vi "Analog Parse Configuration Parameters.vi"(10 "Analog Configuration Parameters":T1) -> (0 "name to assign":string, 1 "physical channels":string, 3 "Maximum Voltage":dbl, 5 "Minimum Voltage":dbl, 7 "Terminal Configuration":i32)   [LabVIEW 2021]
uses:
  Analog Configuration Parameters.ctl
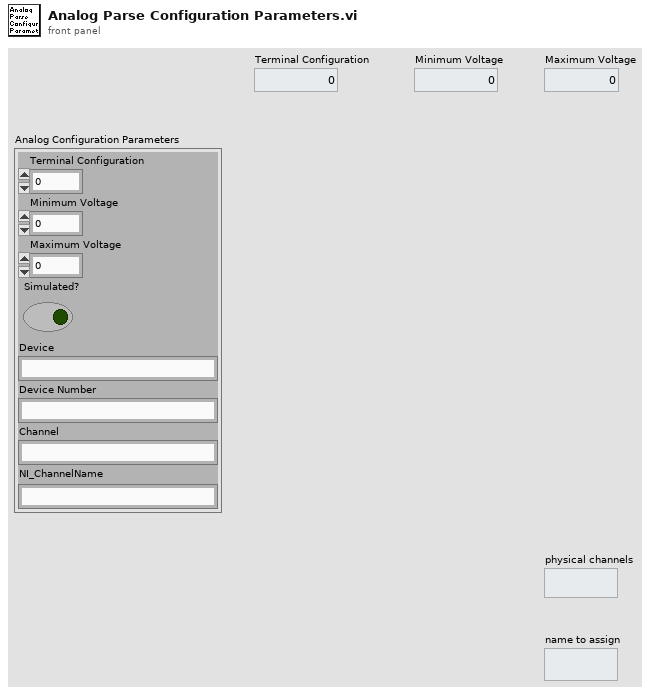
[diagram p1: front panel]
types:
  T1 = typedef "Analog Configuration Parameters.ctl" = cluster{"Terminal Configuration":i32, "Minimum Voltage":dbl, "Maximum Voltage":dbl, "Simulated?":bool, "Device":string, "Device Number":string, "Channel":string, "NI_ChannelName":string}
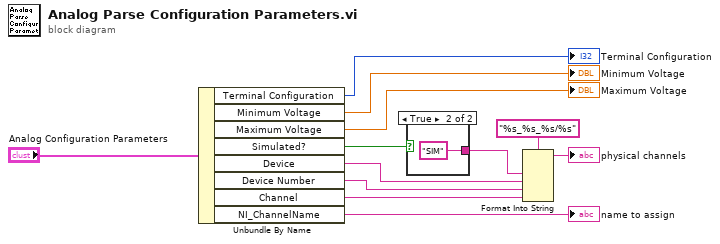
[diagram p0: block diagram]
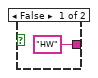
[diagram p2: hidden frame]
diagram:
  n1 = Unbundle By Name("Analog Configuration Parameters") -> ("Terminal Configuration"=→"Terminal Configuration":i32, "Minimum Voltage"=→"Minimum Voltage":dbl, "Maximum Voltage"=→"Maximum Voltage":dbl, "Simulated?"=w2:bool, "Device"=w6:string, "Device Number"=w4:string, "Channel"=w5:string, "NI_ChannelName"=→"name to assign":string)
  n2 = case shown="True" w2 {
    tunnel: ["HW" ("format string") "SIM" ("format string")] -> w1
    frame False {
    }
    frame True {
    }
  }
  n3 = Format Into String(format string="%s_%s_%s/%s", w1, w6, w4, w5) -> (resulting string=→"physical channels":string)  [unwired: 2 in, 1 out]
